vi "Write ER2007 Data File.vi"(0 "PathIn":path=path "C:/ER2005/Data", 1 "Filename":string="Test001.txt", 2 "Header":string[](array[string])=["Date: 07/27/2005", "Time: 19:25", "Filename: C:\\ER2005\\Data\\Test001.dat", "Project: Test File Format Project", "Sample ID: Test Sample", "Rock Type: Hard as a rock", "Fluid Pair: Astair and Rogers", "RW: 11.321", "RW Temp: 23.1", "Frequency: 1000", "Amplitude: 1.00", "DAQ Period (mins): 10", "Length: 5.08", "Diameter: 2.54", "Porosity: 33.33", "Permeability: 8.12", "Elect Spacing: 2.54"], 3 "UnusedColList":i32[](array[numeric]), 4 "DataIn":dbl[](array[numeric])=[1.0, 2.0, 3.0, 4.0, 5.0, 6.0, 7.0, 8.0, 9.0, 10.0, 11.0, 12.0, 13.0, 14.0, 15.0] format="%.3f", 5 "Comment":string, 6 "Function":enum16{"Do Nothing", "Header", "Data"}(ring), 7 "ColHdrText":string[](array[string])=[" Point\t Point\t Point\tEl-Time\t ER 1-2\t ER 1-3\t ER 1-4\t ER 2-3\t F 2-3\t Temp-A\t Temp-B\t  NOP\t   Pc\t  Pdp\t   Pdn\t P-Vol\t  C14\t  C23", "  Flag\t  Date\t  Time\t(Hours)\t(ohm-m)\t(ohm-m)\t(ohm-m)\t(ohm-m)\t  ()  \t(deg-C)\t(deg-C)\t (psig)\t (psig)\t (psid)\t (psig)\t  (ml)\t  (pf)\t  (pf)", "-------\t-------\t-------\t-------\t-------\t-------\t-------\t-------\t-------\t-------\t-------\t-------\t-------\t-------\t-------\t-------\t-------\t-------"], 8 "Check File (F)":bool, 9 "Mark Line":bool, 11 "Mark String":string="   V   ") -> (14 "FilepathOut":path, 19 "OK":bool)   [LabVIEW 2013]
doc: "This vi writes the ER2005 data file that contains all the test data. Required inputs are the path 'PathIn', the name for the file 'Filename', the write function 'Function' and, depending on 'Function', the header information 'Header', and the test data 'Data'. An input is also provided for the column header text 'ColHdrText' that is placed after the header info and before the test data. The test data must be a 1D array. If there are columns in the data that do not need to be placed in the file they should be specified at 'Unused ColList'. Set 'Check File' to TRUE to force a file dialog if the file exists. Boolean 'OK' is TRUE if the file write went OK.\n\nAutoCon, 8/2002 \n\n10/2002 - added shift registers to remember finame between Header & Data\n - modified subvi Append, Replace Cancel or New (see that vi)"
panel:
  in  "Case Constant\n(See Context Help)":bool
  in  "Col Format":string[](array[string])=["%7.2f", "%7.3f", "%7.3f", "%7.3f", "%7.3f", "%7.1f", "%7.1f", "%7.1f", "%7.0f", "%7.2f", "%7.2f", "%7.2f", "%7.2f", "%7.0f", "%7.0f"]
  out "String Out":string
  # "1 = ElapT"
  # "ER 1-2"
  # "ER 1-3"
  # "ER 1-4"
  # "5 = ER 2-3"
  # "F 2-3"
  # "TA"
  # "TB"
  # "NOP"
  # "10 = Pc"
  # "Pdp"
  # "Pdn"
  # "Vol"
  # "C14"
  # "15 = C23"
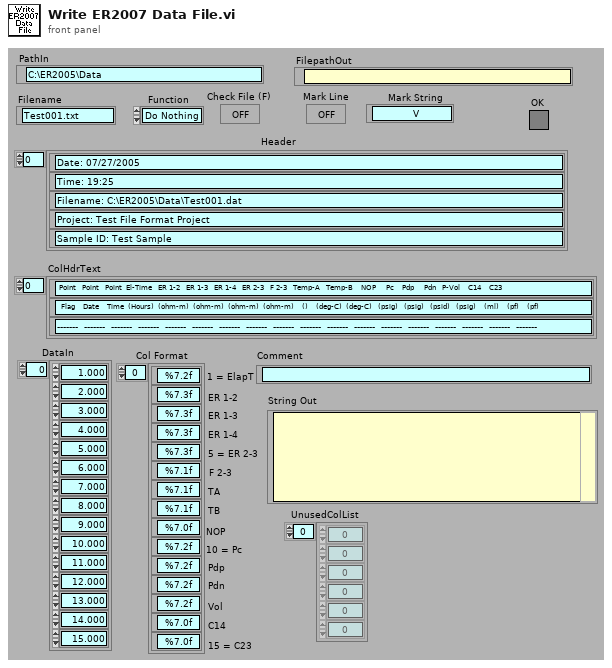
[diagram p1: front panel]
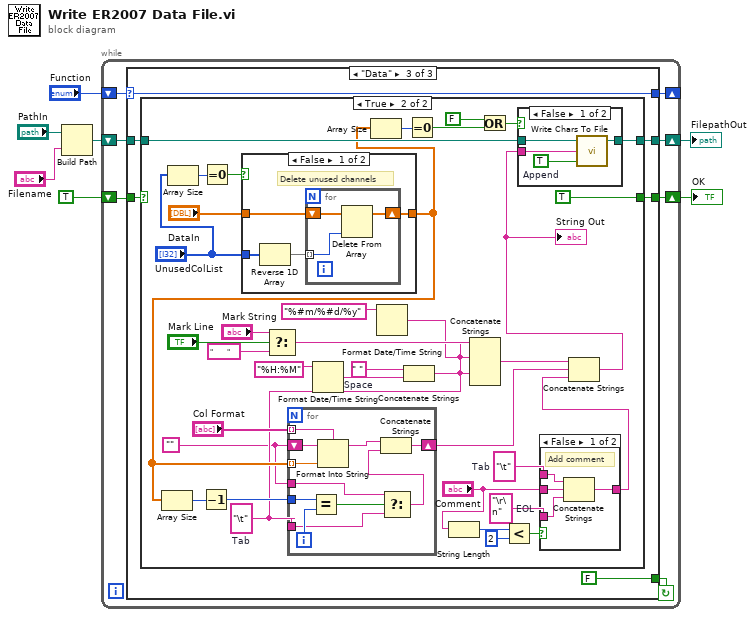
[diagram p0: block diagram]
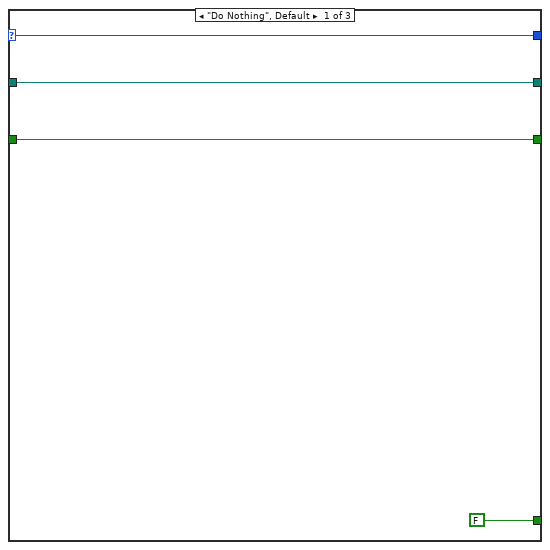
[diagram p2: hidden frame]
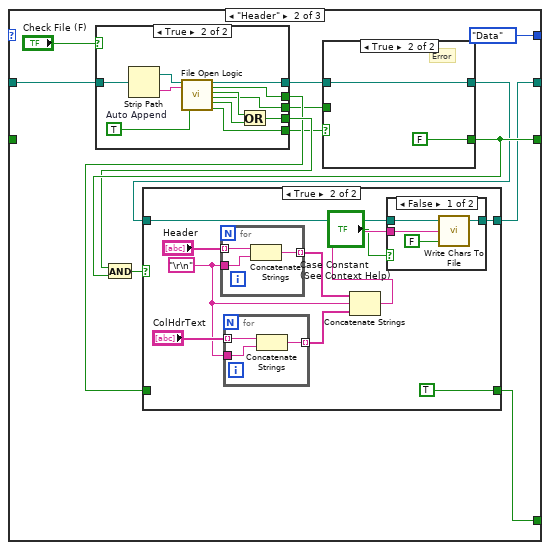
[diagram p3: hidden frame]
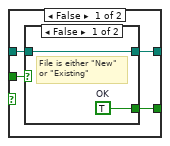
[diagram p4: hidden frame]
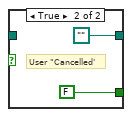
[diagram p5: hidden frame]
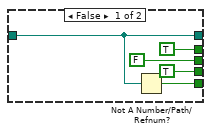
[diagram p6: hidden frame]
diagram:
  n1 = Build Path(base path="PathIn", name or relative path="Filename") -> (appended path=w3:path)
  n2 = while {
    shift-left: w3 -> [w9]
    shift-right: [w8] -> w2
    shift-left: "Function" -> [w12]
    shift-right: [w11] -> _
    shift-left: TRUE -> [w13]
    shift-right: [w14] -> w7
    stop <- w10 continue-if-true
    n3 = case shown="\"Data\"" w12 {
      selector: w12 -> [w15 _ w81]
      tunnel: [w18 w30 w84] -> w8
      tunnel: w9 -> [w18 w19 w85]
      tunnel: [w17 w31 w83] -> w14
      tunnel: w13 -> [w17 _ w86]
      tunnel: [w15 enum16{"Do Nothing", "Header", "Data"}."Data" ("Function") w81] -> w11
      tunnel: [FALSE w28 FALSE] -> w10
      frame "Do Nothing", Default {
      }
      frame "Header" {
        n4 = case shown="True" "Check File (F)" {
          tunnel: w19 -> [w42 w49]
          tunnel: [TRUE w55] -> w26
          tunnel: [TRUE ("AppndOut") w54] -> w25
          tunnel: [FALSE ("CancelOut") w53] -> w23
          tunnel: [w42 w52] -> w22
          tunnel: [w43 w51] -> w20
          frame False {
            n5 = Not A Number/Path/Refnum?(number/path/refnum=w42) -> (NaN/Path/Refnum?=w43:bool)
          }
          frame True {
            w47 = TRUE  # Auto Append
            n6 = Strip Path(path=w49) -> (stripped path=w50:path, name=w48:string)
            n7 = call "File Open Logic.vi"("PathIn"=w50, "Filename"=w48, "Auto Append"=w47) -> ("FullPathOut"=w52:path, "AppndOut"=w54:bool, "ReplOut"=w56:bool, "CancelOut"=w53:bool, "NewOut"=w57:bool, "ErrOut"=w51:bool)  [unwired: 11 in]
            n8 = Or(x=w56, y=w57) -> (x .or. y?=w55:bool)
          }
        }
        n9 = case shown="True" w20 {
          tunnel: [w35 FALSE ("OK")] -> w31
          tunnel: [w34 w41] -> w29
          tunnel: w23 -> [w33 _]
          tunnel: w22 -> [w32 w41]
          frame False {
            n10 = case shown="False" w33 {
              tunnel: w32 -> [w36 _]
              tunnel: [w37 FALSE ("OK")] -> w35
              tunnel: [w36 path ""] -> w34
              frame False {
                w37 = TRUE  # OK
                # "File is either \"New\"\nor \"Existing\""
              }
              frame True {
                # "User \"Cancelled'"
              }
            }
          }
          frame True {
            # "Error"
          }
        }
        n11 = And(x=w26, y=w31) -> (x .and. y?=w27:bool)
        n12 = case shown="True" w27 {
          tunnel: w29 -> [w59 w69]
          tunnel: [w59 w68] -> w30
          tunnel: [w58 TRUE ("AppndOut")] -> w28
          tunnel: w25 -> [w58 _]
          frame False {
            # "Error or file append"
          }
          frame True {
            w60 = "\r\n"
            n13 = for {
              tunnel: "Header" -> [w80] mode=indexing
              tunnel: w60 -> [w79]
              tunnel: [w78] -> w66 mode=indexing
              n14 = Concatenate Strings(w80, w79) -> (w78:string)
            }
            n15 = for {
              tunnel: "ColHdrText" -> [w77] mode=indexing
              tunnel: w60 -> [w76]
              tunnel: [w75] -> w64 mode=indexing
              n16 = Concatenate Strings(w77, w76) -> (w75:string)
            }
            n17 = Concatenate Strings(w66, w60, w64) -> (w63:string)
            n18 = case shown="False" "Case Constant\n(See Context Help)" {
              tunnel: w69 -> [w72 w74]
              tunnel: [w71 w74] -> w68
              tunnel: w63 -> [w70 _]
              frame False {
                n19 = call "Write Chars To File.vi"("append to file? (new file:F)"=FALSE, "character string"=w70, "file path (dialog if empty)"=w72) -> ("new file path (Not A Path if cancelled)"=w71:path)  [unwired: 2 in]
              }
              frame True {
                # "Suppress write"
              }
            }
          }
        }
      }
      frame "Data" {
        n20 = case shown="True" w86 {
          selector: w86 -> [w87 _]
          tunnel: w85 -> [w88 w124]
          tunnel: [w88 w123] -> w84
          tunnel: [w87 TRUE] -> w83
          frame False {
            # "Previous error"
          }
          frame True {
            w92 = "\t"  # Tab
            w93 = "\r\n"  # EOL
            w99 = " "  # Space
            w107 = "\t"  # Tab
            w89 = ""
            n21 = Array Size(array="UnusedColList") -> (size(s)=w116:i32)
            n22 = Equal To 0?(x=w116) -> (x = 0?=w115:bool)
            n23 = case shown="False" w115 {
              tunnel: "DataIn" -> [w145 w149]
              tunnel: [w144 w149] -> w112
              tunnel: "UnusedColList" -> [w143 _]
              frame False {
                # "Delete unused channels"
                n24 = Reverse 1D Array(array=w143) -> (reversed array=w142:i32[])
                n25 = for {
                  shift-right: [w147] -> w144
                  shift-left: w145 -> [w148]
                  tunnel: w142 -> [w146] mode=indexing
                  n26 = Delete From Array(array=w148, index=w146) -> (array with subset deleted=w147:dbl[])  [unwired: 1 in, 1 out]
                }
              }
              frame True {
                # "Nothing to delete"
              }
            }
            n27 = Array Size(array=w112) -> (size(s)=w114:i32)
            n28 = Decrement(x=w114) -> (x-1=w113:i32)
            n29 = Select(t="Mark String", s="Mark Line", f="       ") -> (s? t:f=w108:string)
            n30 = for {
              tunnel: w112 -> [w141] mode=indexing
              shift-right: [w137] -> w105
              shift-left: w89 -> [w140]
              tunnel: "Col Format" -> [w139] mode=indexing
              tunnel: w113 -> [w136]
              tunnel: w89 -> [w132]
              tunnel: w107 -> [w131]
              i -> [w135]
              n31 = Equal?(x=w136, y=w135) -> (x = y?=w134:bool)
              n32 = Format Into String(format string=w139, initial string=w140, w141) -> (resulting string=w138:string)  [unwired: 1 in, 1 out]
              n33 = Select(t=w132, s=w134, f=w131) -> (s? t:f=w133:string)
              n34 = Concatenate Strings(w138, w133) -> (w137:string)
            }
            n35 = Format Date/Time String(time format string (%c)="%H:%M") -> (date/time string=w98:string)  [unwired: 2 in]
            n36 = Array Size(array=w112) -> (size(s)=w119:i32)
            n37 = Format Date/Time String(time format string (%c)="%#m/%#d/%y") -> (date/time string=w103:string)  [unwired: 2 in]
            n38 = Concatenate Strings(w99, w98) -> (w100:string)
            n39 = Equal To 0?(x=w119) -> (x = 0?=w120:bool)
            n40 = String Length(string="Comment") -> (length=w97:i32)
            n41 = Concatenate Strings(w108, w107, w103, w107, w100, w107) -> (w106:string)
            n42 = Or(x=FALSE, y=w120) -> (x .or. y?=w122:bool)
            n43 = Less?(x=w97, y=2) -> (x < y?=w95:bool)
            n44 = case shown="False" w95 {
              tunnel: "Comment" -> [w129 _]
              tunnel: w93 -> [w128 w130]
              tunnel: w92 -> [w127 _]
              tunnel: [w126 w130] -> w90
              frame False {
                # "Add comment"
                n45 = Concatenate Strings(w127, w129, w128) -> (w126:string)
              }
              frame True {
                # "No comment"
              }
            }
            n46 = Concatenate Strings(w106, w105, w90) -> (w91:string)
            "String Out" <- w91
            n47 = case shown="False" w122 {
              tunnel: w124 -> [w153 w154]
              tunnel: [w152 w154] -> w123
              tunnel: w91 -> [w151 _]
              frame False {
                w150 = TRUE  # Append
                n48 = call "Write Chars To File.vi"("append to file? (new file:F)"=w150, "character string"=w151, "file path (dialog if empty)"=w153) -> ("new file path (Not A Path if cancelled)"=w152:path)  [unwired: 2 in]
              }
              frame True {
                # "Suppress write"
              }
            }
          }
        }
      }
    }
  }
  "FilepathOut" <- w2
  "OK" <- w7
